vi "compute_slopes_on_image_starter.vi"() -> ()   [LabVIEW 2020]
uses:
  Image.lvclass
  HasoSlopes.lvclass
  Point2D.ctl
panel:
  out "Y Slopes":sgl[][](graph)
  in  "Image file name":string="Data\\data_image.himg"
  in  "Haso configuration file name":string="Data\\config_file_haso.dat"
  in  "Output file name":string="Data\\data_phase_computation_example.has"
  out "X Slopes":sgl[][](graph)
  out "error out":errorcluster
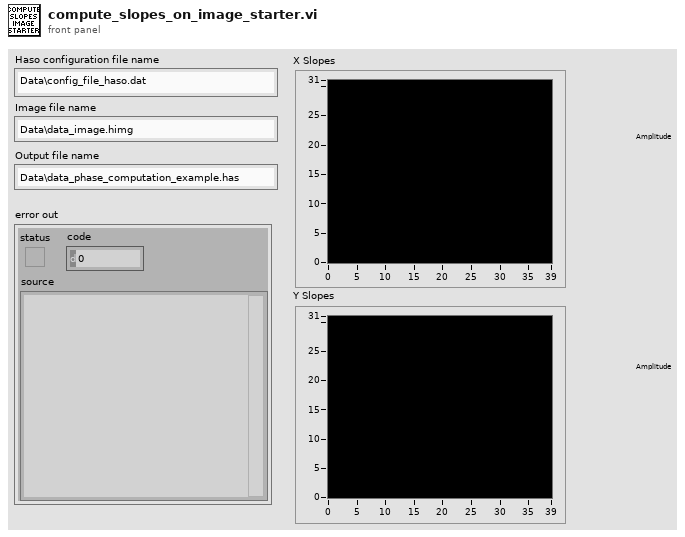
[diagram p1: front panel]
types:
  T1 = typedef "Point2D.ctl" = cluster{"X":u32, "Y":u32}
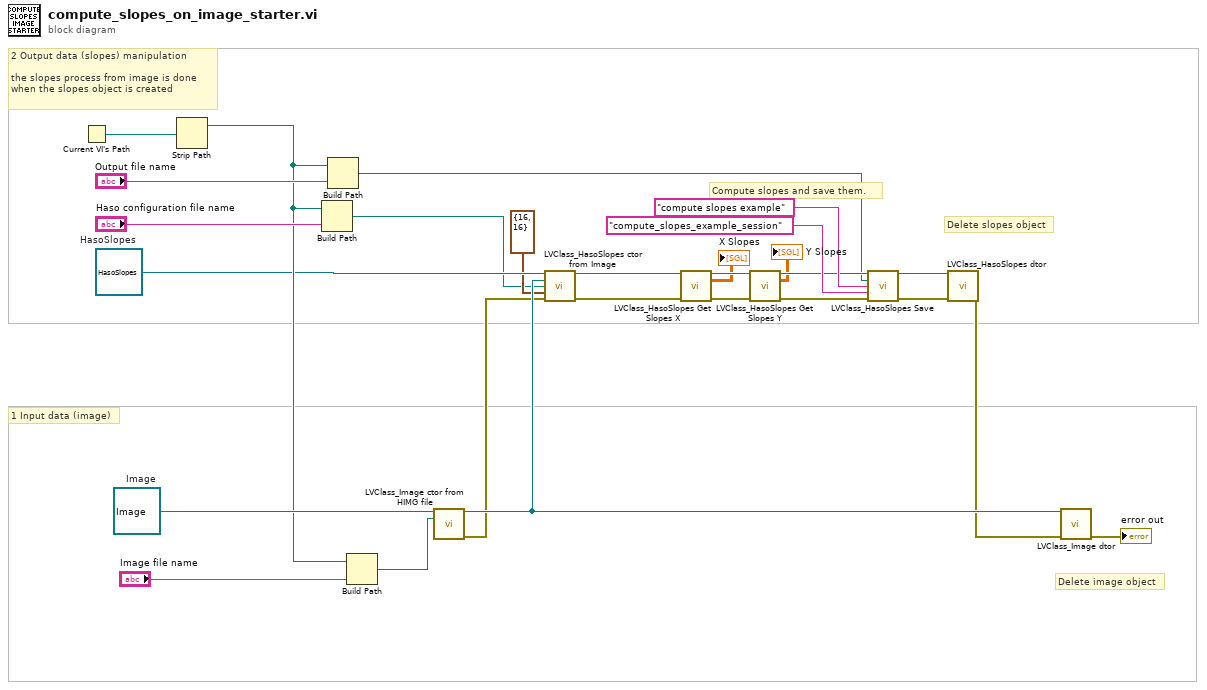
[diagram p0: block diagram]
diagram:
  w12 = refnum<class "HasoSlopes.lvclass"> refnum  # HasoSlopes
  w27 = refnum<class "Image.lvclass"> refnum  # Image
  # "Delete image object"
  # "2 Output data (slopes) manipulation\n\nthe slopes process from image is done \nwhen the slopes object is created"
  # "1 Input data (image)"
  # "Delete slopes object"
  # "Compute slopes and save them."
  n1 = Current VI's Path() -> (path=w22:path)
  n2 = Strip Path(path=w22) -> (stripped path=w19:path)  [unwired: 1 out]
  n3 = Build Path(base path=w19, name or relative path="Haso configuration file name") -> (appended path=w4:path)
  n4 = Build Path(base path=w19, name or relative path="Output file name") -> (appended path=w5:path)
  n5 = Build Path(base path=w19, name or relative path="Image file name") -> (appended path=w3:path)
  n6 = call "LVClass_Image ctor from HIMG file.vi"("Image in"=w27, "Path to image file"=w3) -> ("Image out"=w11:refnum<class "Image.lvclass">, "error out"=w9:errorcluster)  [unwired: 12 in]
  n7 = call "LVClass_HasoSlopes ctor from Image.vi"("HasoSlopes in"=w12, "Image.lvclass"=w11, "Haso configuration file"=w4, "start subpupil"=T1 {"X"=16, "Y"=16} ("ImageSize"), "error in (no error)"=w9) -> ("HasoSlopes out"=w8:refnum<class "HasoSlopes.lvclass">, "error out"=w6:errorcluster)  [unwired: 9 in]
  n8 = call "LVClass_HasoSlopes Get Slopes X.vi"("HasoSlopes in"=w8, "error in (no error)"=w6) -> ("HasoSlopes out"=w18:refnum<class "HasoSlopes.lvclass">, "Slopesx"=→"X Slopes":sgl[][], "error out"=w17:errorcluster)  [unwired: 11 in]
  n9 = call "LVClass_HasoSlopes Get Slopes Y.vi"("HasoSlopes in"=w18, "error in (no error)"=w17) -> ("HasoSlopes out"=w16:refnum<class "HasoSlopes.lvclass">, "Slopesy"=→"Y Slopes":sgl[][], "error out"=w13:errorcluster)  [unwired: 11 in]
  n10 = call "LVClass_HasoSlopes Save.vi"("HasoSlopes in"=w16, "path"=w5, "comments"="compute slopes example", "session"="compute_slopes_example_session", "error in (no error)"=w13) -> ("HasoSlopes out"=w7:refnum<class "HasoSlopes.lvclass">, "error out"=w2:errorcluster)  [unwired: 9 in]
  n11 = call "LVClass_HasoSlopes dtor.vi"("HasoSlopes in"=w7, "error in (no error)"=w2) -> ("error out"=w1:errorcluster)  [unwired: 12 in, 1 out]
  n12 = call "LVClass_Image dtor.vi"("Image in"=w11, "error in (no error)"=w1) -> ("error out"=→"error out":errorcluster)  [unwired: 12 in, 1 out]
